vi "Numeric Array to String.vi"(10 "List Data":dbl[](array[numeric])) -> (2 "Result String":string)   [LabVIEW 2012, in "Keysight B2980 Series.lvlib"]
doc: "Parse a numeric array into a comma separated string which can be recognized by SCPI commads."
uses:
  Keysight B2980 Series.lvlib
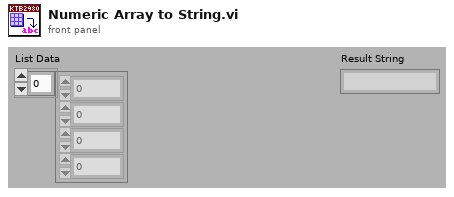
[diagram p1: front panel]
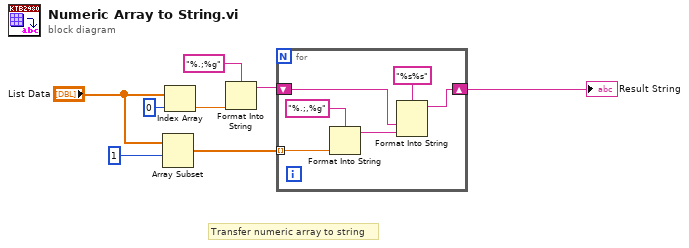
[diagram p0: block diagram]
diagram:
  # "Transfer numeric array to string"
  n1 = Array Subset(array="List Data", index=1) -> (w8:dbl[])  [unwired: 1 in]
  n2 = Index Array(array="List Data", index=0) -> (element=w4:dbl)
  n3 = Format Into String(format string="%.;%g", w4) -> (resulting string=w3:string)  [unwired: 2 in, 1 out]
  n4 = for {
    tunnel: w8 -> [w14] mode=indexing
    shift-right: [w12] -> w2
    shift-left: w3 -> [w11]
    n5 = Format Into String(format string="%.;,%g", w14) -> (resulting string=w10:string)  [unwired: 2 in, 1 out]
    n6 = Format Into String(format string="%s%s", w11, w10) -> (resulting string=w12:string)  [unwired: 2 in, 1 out]
  }
  "Result String" <- w2
